vi "GetTimeDifferenceFromHRCounter.vi"(1 "StopCounter":i64, 2 "StartCounter":i64) -> (0 "difference time":dbl)   [LabVIEW 2009]
uses:
  kernel32.dll
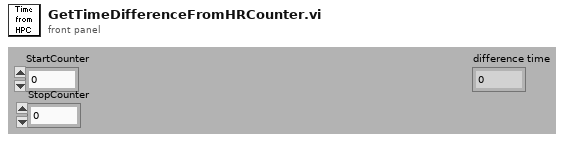
[diagram p1: front panel]
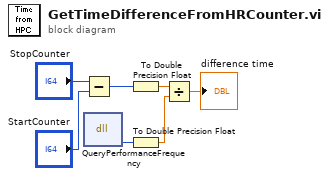
[diagram p0: block diagram]
diagram:
  n1 = Subtract(x="StopCounter", y="StartCounter") -> (x-y=w5:i64)
  n2 = dll-call lib="kernel32.dll" fn="QueryPerformanceFrequency"() -> ("PerformanceFrequency"=w1:i64)  [unwired: 3 in, 4 out]
  n3 = To Double Precision Float(number=w5) -> (double precision float=w4:dbl)
  n4 = To Double Precision Float(number=w1) -> (double precision float=w3:dbl)
  n5 = Divide(x=w4, y=w3) -> (x/y=→"difference time":dbl)
